vi "XIPIN_RLDRAM3_PHY_IP_1_1.vi"   [LabVIEW 2017]
doc: "PHY for RLD3 interfaces for Ultrascale Architecture\n------------------------------------\n<b>Need License</b> : No"
uses:
  <vilib>/rvi/XilinxIP/XIPIN_XNode/niFpgaXIPIN.xnode
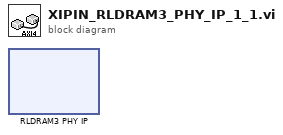
[diagram p0: block diagram]
diagram:
  n1 = xnode ("RLDRAM3 PHY IP")() -> ()
